vi "Copy Method VI.vi"(8 "error in (no error)":errorcluster, 9 "DVR API Suffix":string=" API", 10 "DVR API Directory Path":path, 11 "Class Method Path":path) -> (0 "error out":errorcluster, 3 "DVR Method Path Out":path)   [LabVIEW 2016, in "SLL Scripting.lvlib" / "SLL Class DVR API Generator.lvlib"]
uses:
  SLL Class DVR API Generator.lvlib
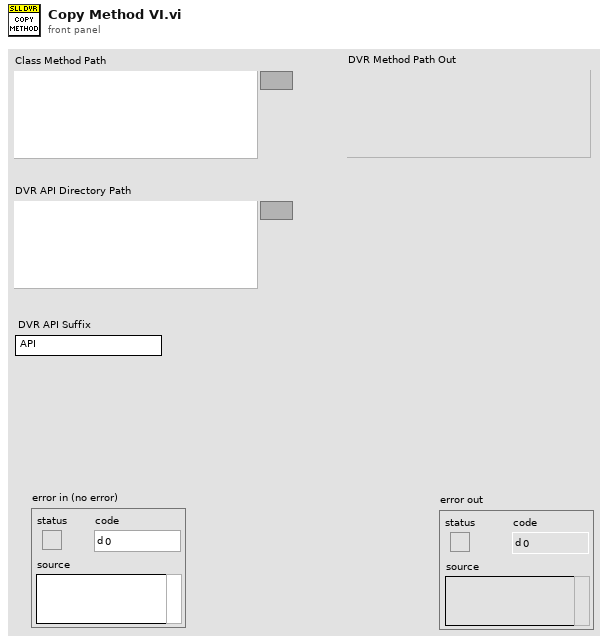
[diagram p1: front panel]
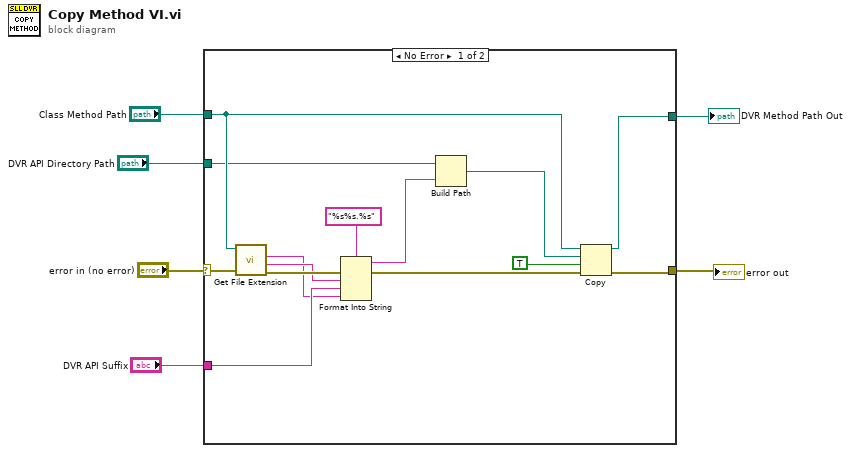
[diagram p0: block diagram]
diagram:
  n1 = case shown="No Error" "error in (no error)" {
    selector: "error in (no error)" -> [w19 w21]
    tunnel: [w9 w21] -> w5
    tunnel: "Class Method Path" -> [w18 _]
    tunnel: "DVR API Directory Path" -> [w12 _]
    tunnel: "DVR API Suffix" -> [w14 _]
    tunnel: [w7 _] -> w1
    frame No Error {
      n2 = call <vilib>:"Get File Extension.vi"("error in (no error)"=w19, "file"=w18) -> ("error out"=w17:errorcluster, "filename without extension"=w15:string, "lowercase file extension"=w13:string)  [unwired: 5 in, 2 out]
      n3 = Format Into String(format string="%s%s.%s", error in=w17, w15, w14, w13) -> (resulting string=w11:string, error out=w10:errorcluster)  [unwired: 1 in]
      n4 = Build Path(base path=w12, name or relative path=w11) -> (appended path=w8:path)
      n5 = Copy(8:w10, 9:TRUE ("overwrite (F)"), 10:w8, 11:w18) -> (0:w9:errorcluster, 3:w7:path)  [unwired: 1 in, 1 out]
    }
    frame Error {
    }
  }
  "error out" <- w5
  "DVR Method Path Out" <- w1
